vi "FSM.vi"() -> ()   [LabVIEW 2018]
panel:
  in  "Restart":bool
  in  "Start Running":bool
  in  "Reset":bool
  out "Initializing":bool
  out "Running":bool
  in  "Start Initializing":bool
  in  "stop":bool
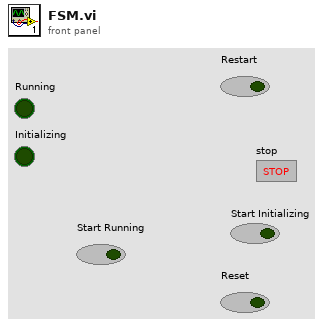
[diagram p1: front panel]
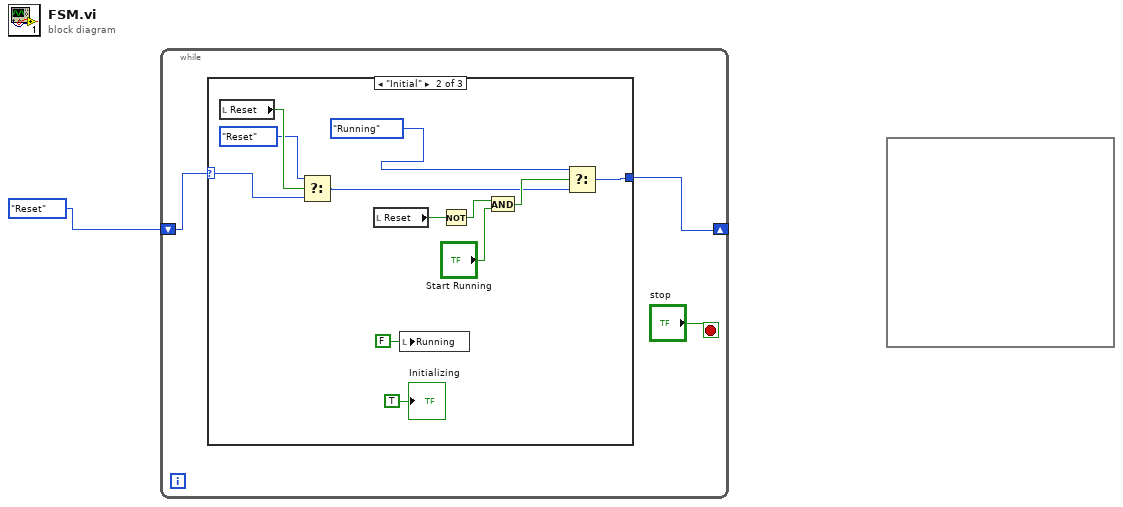
[diagram p0: block diagram]
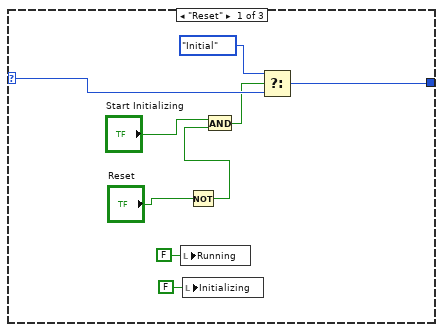
[diagram p2: hidden frame]
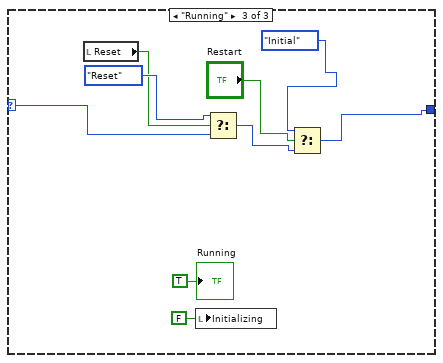
[diagram p3: hidden frame]
diagram:
  n1 = while {
    shift-right: [w3] -> _
    shift-left: enum16{"Reset", "Initial", "Running"}."Reset" -> [w2]
    stop <- "stop" stop-if-true
    n2 = case shown="\"Initial\"" w2 {
      selector: w2 -> [w12 w14 w31]
      tunnel: [w11 w23 w33] -> w3
      frame "Reset" {
        n3 = local write "Running"(FALSE ("Running")) -> ()
        n4 = local write "Initializing"(FALSE ("Initializing")) -> ()
        n5 = Not(x="Reset") -> (.not. x?=w9:bool)
        n6 = And(x="Start Initializing", y=w9) -> (x .and. y?=w7:bool)
        n7 = Select(t=enum16{"Reset", "Initial", "Running"}."Initial", s=w7, f=w12) -> (s? t:f=w11:enum16{"Reset", "Initial", "Running"})
      }
      frame "Initial" {
        n8 = local read "Reset"() -> (w16:bool)
        n9 = Select(t=enum16{"Reset", "Initial", "Running"}."Reset", s=w16, f=w14) -> (s? t:f=w17:enum16{"Reset", "Initial", "Running"})
        n10 = local read "Reset"() -> (w25:bool)
        n11 = local write "Running"(FALSE ("Running")) -> ()
        n12 = Not(x=w25) -> (.not. x?=w18:bool)
        n13 = And(x=w18, y="Start Running") -> (x .and. y?=w20:bool)
        n14 = Select(t=enum16{"Reset", "Initial", "Running"}."Running", s=w20, f=w17) -> (s? t:f=w23:enum16{"Reset", "Initial", "Running"})
        "Initializing" <- TRUE ("Initializing")
      }
      frame "Running" {
        n15 = local read "Reset"() -> (w29:bool)
        n16 = local write "Initializing"(FALSE ("Initializing")) -> ()
        n17 = Select(t=enum16{"Reset", "Initial", "Running"}."Reset", s=w29, f=w31) -> (s? t:f=w28:enum16{"Reset", "Initial", "Running"})
        n18 = Select(t=enum16{"Reset", "Initial", "Running"}."Initial", s="Restart", f=w28) -> (s? t:f=w33:enum16{"Reset", "Initial", "Running"})
        "Running" <- TRUE ("Running")
      }
    }
  }
  n19 = formula code=""() -> ()
